vi "Initialize Attributes.vi"(8 "error in (no error)":errorcluster, 10 "Attribute Data":variant, 11 "KIT-QA in":refnum<class "KIT-QA.lvclass">) -> (0 "error out":errorcluster, 2 "Found?":bool, 3 "KIT-QA out":refnum<class "KIT-QA.lvclass">)   [LabVIEW 2015, in "KIT-QA.lvlib" / "KIT-QA.lvclass"]
doc: "Initialize object attribute.\n\nUnique resources should be allocated elsewhere!"
uses:
  KIT-QA.lvclass
  CSPP_Core/Actors/CS++BaseActor/CS++BaseActor.lvclass/CS++BaseActor.ctl
  KIT-QA.lvclass/KIT-QA.ctl
  CSPP_Core/Actors/CS++GUIActor/CS++GUIActor.lvclass
  CSPP_Core/Classes/CS++BaseClasses/Factory/CS++Factory.lvclass
  CSPP_Core/Libraries/Utilities/CS++Utilities.lvlib
  CSPP_Core/Actors/CS++BaseActor/CS++BaseActor.lvclass
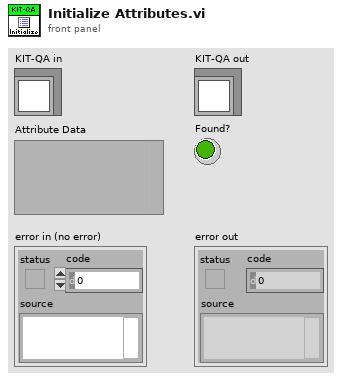
[diagram p1: front panel]
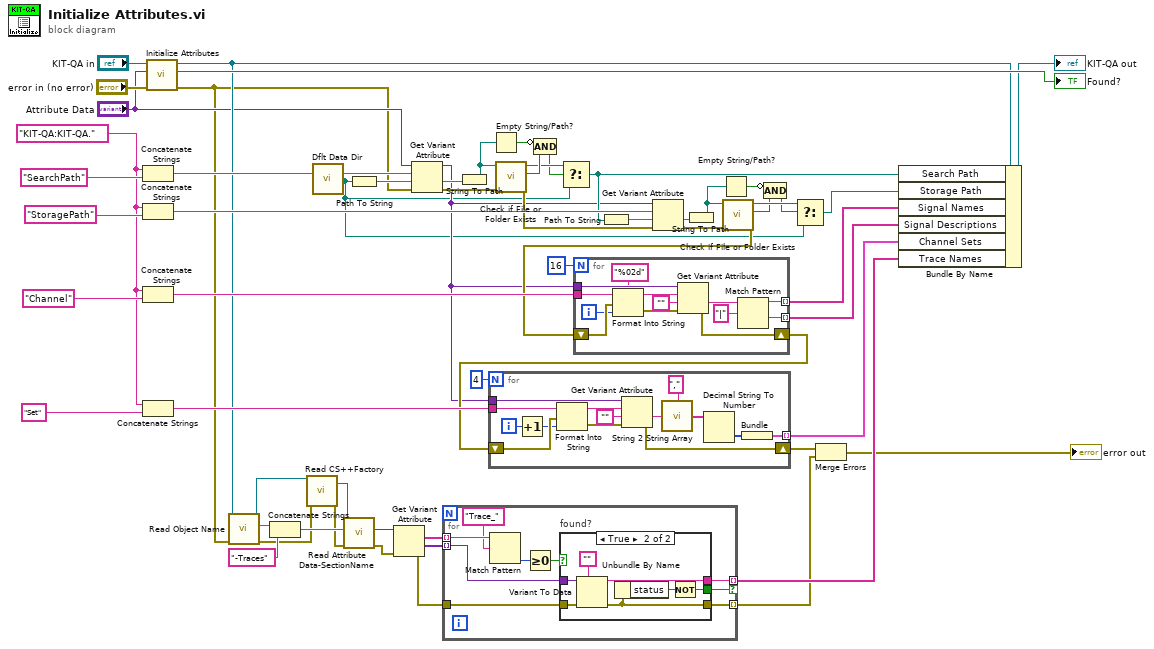
[diagram p0: block diagram]
diagram:
  w17 = "KIT-QA:KIT-QA."
  n1 = Concatenate Strings(w17, "SearchPath") -> (w56:string)
  n2 = Concatenate Strings(w17, "StoragePath") -> (w34:string)
  n3 = Concatenate Strings(w17, "Channel") -> (w48:string)
  n4 = Concatenate Strings(w17, "Set") -> (w42:string)
  n5 = call-parent "Initialize Attributes.vi"("error in (no error)"="error in (no error)", "Attribute Data"="Attribute Data", "CS++GUIActor in"="KIT-QA in") -> ("error out"=w1:errorcluster, "Found?"=→"Found?":bool, "CS++GUIActor out"=w11:refnum<class "KIT-QA.lvclass">)  [unwired: 6 in]
  n6 = call "Read Object Name.vi"("error in (no error)"=w1, "CS++BaseActor in"=w11) -> ("error out"=w6:errorcluster, "Object Name"=w10:string, "CS++BaseActor out"=w9:refnum<class "KIT-QA.lvclass">)  [unwired: 7 in]
  n7 = Concatenate Strings(w10, "-Traces" ("string")) -> (w8:string)
  n8 = call "Read CS++Factory.vi"("error in (no error)"=w6, "CS++BaseActor in"=w9) -> ("error out"=w5:errorcluster, "CS++Factory"=w12:refnum<class "CS++Factory.lvclass">)  [unwired: 7 in, 1 out]
  n9 = call <vilib>:"Dflt Data Dir.vi"() -> ("App:Default Data Directory"=w20:path)
  n10 = call-dynamic "Read Attribute Data-SectionName.vi"("error in (no error)"=w5, "Object Name"=w8, "CS++Factory in"=w12) -> ("error out"=w2:errorcluster, "Attribute Data"=w3:variant)  [unwired: 6 in, 1 out]
  n11 = Path To String(path=w20) -> (string=w55:string)
  n12 = Get Variant Attribute(Variant=w3, error in=w2) -> (names=w19:string[], values=w18:variant[], error out=w16:errorcluster)  [unwired: 2 in, 1 out]
  n13 = Get Variant Attribute(Variant="Attribute Data", name=w56, default value (empty Variant)=w55, error in=w1) -> (duplicate Variant=w28:variant, value=w53:string, error out=w47:errorcluster)  [unwired: 1 out]
  n14 = for {
    tunnel: w19 -> [w69] mode=indexing
    tunnel: w18 -> [w66] mode=indexing
    tunnel: [w65] -> w15 mode=indexing if=w62
    tunnel: w16 -> [w64]
    tunnel: [w61] -> w13 mode=indexing
    n15 = Match Pattern(string=w69, regular expression="Trace_") -> (offset past match=w67:i32)  [unwired: 1 in, 3 out]
    n16 = Greater Or Equal To 0?(x=w67) -> (x >= 0?=w63:bool)
    n17 = case "found?" shown="True" w63 {
      tunnel: w66 -> [_ w77]
      tunnel: [_ w75] -> w65
      tunnel: w64 -> [w70 w74]
      tunnel: [_ w72] -> w62
      tunnel: [w70 w71] -> w61
      frame False {
      }
      frame True {
        n18 = Variant To Data(error in=w74, type="", Variant=w77) -> (data=w75:string, error out=w71:errorcluster)
        n19 = Unbundle By Name(w71) -> ("status"=w73:bool)
        n20 = Not(x=w73) -> (.not. x?=w72:bool)
      }
    }
  }
  n21 = String To Path(string=w53) -> (path=w27:path)
  n22 = Empty String/Path?(string/path=w27) -> (empty?=w25:bool)
  n23 = call <vilib>:"Check if File or Folder Exists.vi"("error in (no error)"=w47, "path"=w27) -> ("error out"=w31:errorcluster, "file or folder exists?"=w52:bool, "dup path"=w51:path)  [unwired: 7 in]
  n24 = Compound Arithmetic op=AND(invert w25, w52) -> (w26:bool)
  n25 = Select(t=w51, s=w26, f=w20) -> (s? t:f=w32:path)
  n26 = Path To String(path=w32) -> (string=w35:string)
  n27 = Get Variant Attribute(Variant=w28, name=w34, default value (empty Variant)=w35, error in=w31) -> (value=w36:string, error out=w38:errorcluster)  [unwired: 2 out]
  n28 = String To Path(string=w36) -> (path=w23:path)
  n29 = Empty String/Path?(string/path=w23) -> (empty?=w24:bool)
  n30 = call <vilib>:"Check if File or Folder Exists.vi"("error in (no error)"=w38, "path"=w23) -> ("error out"=w30:errorcluster, "file or folder exists?"=w22:bool, "dup path"=w37:path)  [unwired: 7 in]
  n31 = for {
    N: 16 -> [_]
    tunnel: w28 -> [w90]
    tunnel: w48 -> [w89]
    tunnel: [w81] -> w46 mode=indexing
    tunnel: [w80] -> w45 mode=indexing
    shift-right: [w79] -> w41
    shift-left: w30 -> [w86]
    i -> [w78]
    n32 = Format Into String(format string="%02d", initial string=w89, error in=w86, w78) -> (resulting string=w87:string, error out=w85:errorcluster)
    n33 = Get Variant Attribute(Variant=w90, name=w87, default value (empty Variant)="", error in=w85) -> (value=w83:string, error out=w79:errorcluster)  [unwired: 2 out]
    n34 = Match Pattern(string=w83, regular expression="|") -> (before substring=w81:string, after substring=w80:string)  [unwired: 1 in, 2 out]
  }
  n35 = for {
    N: 4 -> [_]
    tunnel: w28 -> [w104]
    tunnel: w42 -> [w103]
    shift-right: [w98] -> w40
    shift-left: w41 -> [w101]
    tunnel: [w92] -> w39 mode=indexing
    i -> [w95]
    n36 = Increment(x=w95) -> (x+1=w91:i32)
    n37 = Format Into String(initial string=w103, error in=w101, w91) -> (resulting string=w102:string, error out=w100:errorcluster)  [unwired: 1 in]
    n38 = Get Variant Attribute(Variant=w104, name=w102, default value (empty Variant)="", error in=w100) -> (value=w97:string, error out=w98:errorcluster)  [unwired: 2 out]
    n39 = call "String 2 String Array.vi"("String"=w97, "Delimiter (\",\")"="," ("Delimiter (\",\")")) -> ("Substrings"=w94:string[])
    n40 = Decimal String To Number(string=w94) -> (number=w93:i32[])  [unwired: 2 in, 1 out]
    n41 = Bundle(w93) -> (w92:cluster{i32[]})  [unwired: 1 in]
  }
  n42 = Compound Arithmetic op=AND(invert w24, w22) -> (w21:bool)
  n43 = Select(t=w37, s=w21, f=w20) -> (s? t:f=w29:path)
  n44 = Merge Errors(w40, w13) -> (→"error out":errorcluster)
  n45 = Bundle By Name(cluster=w11, "Search Path"=w32, "Storage Path"=w29, "Signal Names"=w46, "Signal Descriptions"=w45, "Channel Sets"=w39, "Trace Names"=w15) -> (→"KIT-QA out":refnum<class "KIT-QA.lvclass">)
